vi "configureAcquisition.vi"(6 "imagePaths":path[](array[path]), 7 "saveImages?":bool, 8 "error in (no error)":errorcluster, 9 "number of Images":i32, 10 "CameraSettings":refnum<class "CamaraSettings.lvclass">, 11 "Pixelfly in":refnum<class "PixelflySA.lvclass">) -> (0 "error out":errorcluster, 3 "Pixelfly out":refnum<class "PixelflySA.lvclass">)   [LabVIEW 2009, in "PixelflySA.lvclass"]
uses:
  PixelflySA.lvclass
  Tools/CameraSettings/CamaraSettings.lvclass
  Tools/CameraSettings/PixelFlySettings/PixelflySettings.lvclass
  PixelflySA.lvclass/PixelflySA.ctl
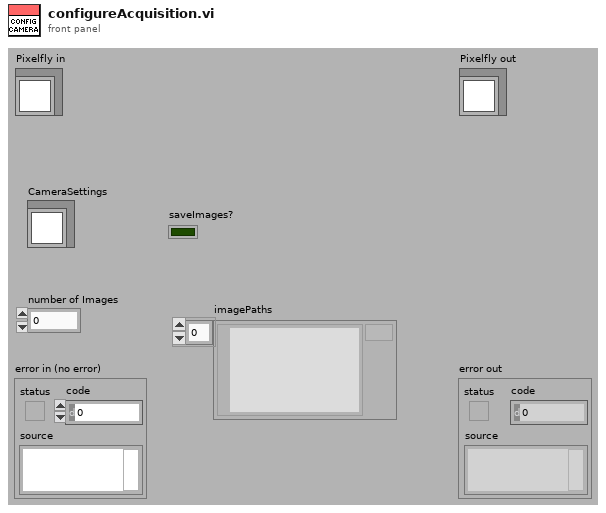
[diagram p1: front panel]
types:
  T1 = cluster{"ccdxsize":i32, "ccdy":i32, "pictx":i32, "picty":i32, "bitspixel":i32}
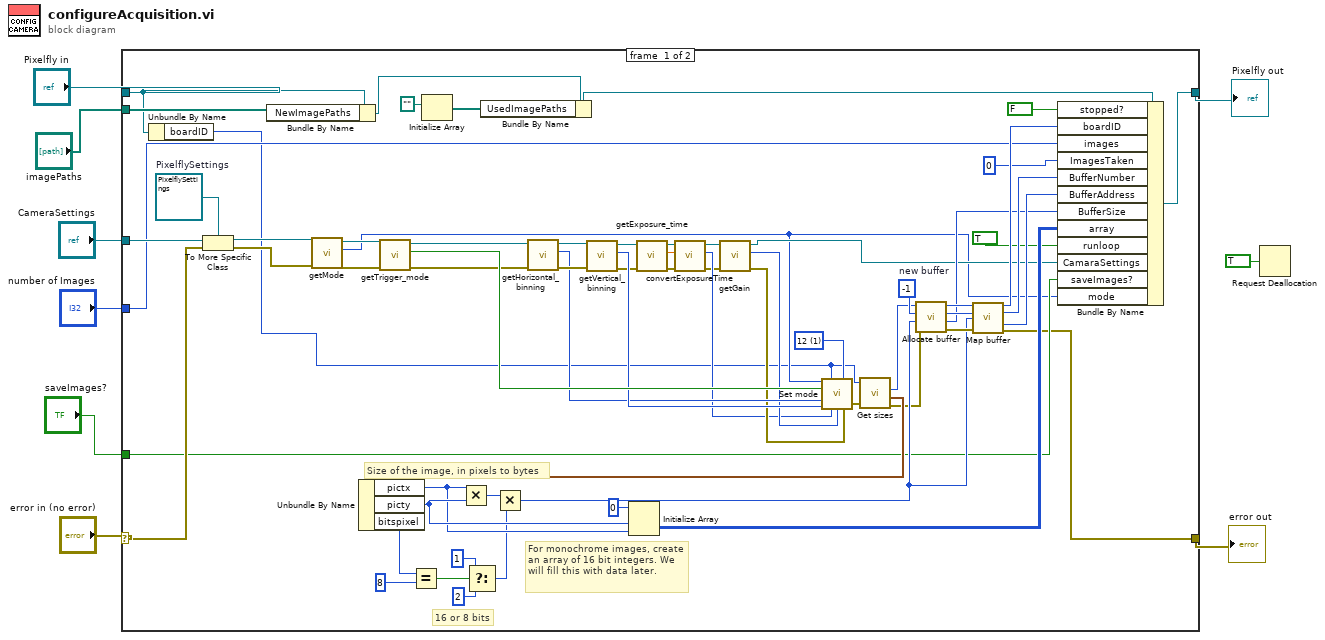
[diagram p0: block diagram]
diagram:
  n1 = case shown="No Error" "error in (no error)" {
    selector: "error in (no error)" -> [w72 w75]
    tunnel: "Pixelfly in" -> [w24 w76]
    tunnel: [w17 w76] -> w5
    tunnel: [w16 w75] -> w4
    tunnel: "CameraSettings" -> [w74 _]
    tunnel: "number of Images" -> [w40 _]
    tunnel: "imagePaths" -> [w25 _]
    tunnel: "saveImages?" -> [w18 _]
    frame #0 {
      w55 = 1 items=["8", "12"] ("bits/pixel")
      w57 = -1  # new buffer
      w73 = refnum<class "PixelflySettings.lvclass"> refnum  # PixelflySettings
      # "16 or 8 bits"
      # "For monochrome images, create an array of 16 bit integers. We will fill this with data later."
      # "Size of the image, in pixels to bytes"
      n2 = Unbundle By Name(w24) -> ("boardID"=w11:i32)
      n3 = To More Specific Class(target class=w73, reference=w74, error in=w72) -> (specific class reference=w54:refnum<class "PixelflySettings.lvclass">, error out=w14:errorcluster)
      n4 = Bundle By Name(cluster=w24, "NewImagePaths"=w25) -> (w23:refnum<class "PixelflySA.lvclass">)
      n5 = call "getMode.vi"("error in (no error)"=w14, "PixelflySettings in"=w54) -> ("error out"=w52:errorcluster, "mode"=w15:u16, "PixelflySettings out"=w53:refnum<class "PixelflySettings.lvclass">)  [unwired: 7 in]
      n6 = call "getTrigger_mode.vi"("error in (no error)"=w52, "PixelflySettings in"=w53) -> ("error out"=w20:errorcluster, "trigger_mode"=w51:bool, "PixelflySettings out"=w50:refnum<class "PixelflySettings.lvclass">)  [unwired: 7 in]
      n7 = Initialize Array(path "") -> (w21:path[])  [unwired: 1 in]
      n8 = Bundle By Name(cluster=w23, "UsedImagePaths"=w21) -> (w22:refnum<class "PixelflySA.lvclass">)
      n9 = call "getHorizontal_binning.vi"("error in (no error)"=w20, "PixelflySettings in"=w50) -> ("error out"=w48:errorcluster, "horizontal_binning"=w46:enum16{"1", "2"}, "PixelflySettings out"=w49:refnum<class "PixelflySettings.lvclass">)  [unwired: 7 in]
      n10 = call "getVertical_binning.vi"("error in (no error)"=w48, "PixelflySettings in"=w49) -> ("error out"=w44:errorcluster, "vertical_binning"=w47:enum16{"1", "2"}, "PixelflySettings out"=w45:refnum<class "PixelflySettings.lvclass">)  [unwired: 7 in]
      n11 = call "getExposure_time.vi"("error in (no error)"=w44, "PixelflySettings in"=w45) -> ("error out"=w30:errorcluster, "exposure_time"=w33:dbl, "PixelflySettings out"=w34:refnum<class "PixelflySettings.lvclass">)  [unwired: 7 in]
      n12 = call "convertExposureTime.vi"("error in (no error)"=w30, "time s"=w33, "PixelflySettings in"=w34) -> ("error out"=w31:errorcluster, "exposureTime"=w32:i32, "PixelflySettings out"=w29:refnum<class "PixelflySettings.lvclass">)  [unwired: 6 in]
      n13 = call "getGain.vi"("error in (no error)"=w31, "PixelflySettings in"=w29) -> ("error out"=w42:errorcluster, "gain"=w43:enum16{"Low", "High"}, "PixelflySettings out"=w19:refnum<class "PixelflySettings.lvclass">)  [unwired: 7 in]
      n14 = call <instrlib>:"Set mode.vi"("Exposure mode"=w15, "Handle in"=w11, "bits/pixel"=w55, "trigger"=w51, "H bin"=w46, "V bin"=w47, "exp time"=w32, "gain"=w43, "error in (no error)"=w42) -> ("error out"=w13:errorcluster)  [unwired: 6 in]
      n15 = call <instrlib>:"Get sizes.vi"("Handle in"=w11, "error in (no error)"=w13) -> ("Handle out"=w10:i32, "Picture parameters"=w66:T1, "error out"=w12:errorcluster)  [unwired: 1 in, 1 out]
      n16 = Unbundle By Name(w66) -> ("pictx"=w63:i32, "picty"=w64:i32, "bitspixel"=w65:i32)
      n17 = Equal?(x=w65, y=8) -> (x = y?=w62:bool)
      n18 = Multiply(x=w63, y=w64) -> (x*y=w68:i32)
      n19 = Select(t=1, s=w62, f=2) -> (s? t:f=w59:i32)
      n20 = Multiply(x=w68, y=w59) -> (x*y=w58:i32)
      n21 = Initialize Array(u16 0 ("16 bit integers"), w64, w63) -> (w36:u16[][])
      n22 = call <instrlib>:"Allocate buffer.vi"("error in (no error)"=w12, "Size request"=w58, "Buffer request"=w57, "Handle in"=w10) -> ("error out"=w70:errorcluster, "Size"=w37:i32, "Buffer number"=w56:i32, "Handle out"=w71:i32)
      n23 = call <instrlib>:"Map buffer.vi"("Handle in"=w71, "Buffer in"=w56, "size"=w58, "error in (no error)"=w70) -> ("Handle out"=w41:i32, "Buffer number"=w39:i32, "Buffer address"=w38:i32, "error out"=w16:errorcluster)  [unwired: 8 in]
      n24 = Bundle By Name(cluster=w22, "stopped?"=FALSE, "boardID"=w41, "images"=w40, "ImagesTaken"=0, "BufferNumber"=w39, "BufferAddress"=w38, "BufferSize"=w37, "array"=w36, "runloop"=TRUE, "CamaraSettings"=w19, "saveImages?"=w18, "mode"=w15) -> (w17:refnum<class "PixelflySA.lvclass">)
    }
    frame #1 {
    }
  }
  "error out" <- w4
  "Pixelfly out" <- w5
  n25 = Request Deallocation(TRUE ("flag")) -> ()
